vi "encodeArrayByte.vi"(8 "error in (no error)":errorcluster, 11 "Byte Array":u8[](array[numeric]) format="%.0x") -> (0 "error out":errorcluster, 3 "MessagePack":u8[](array[numeric]) format="%.0x")   [LabVIEW 2015, in "MsgPack.lvlib"]
uses:
  MsgPack.lvlib
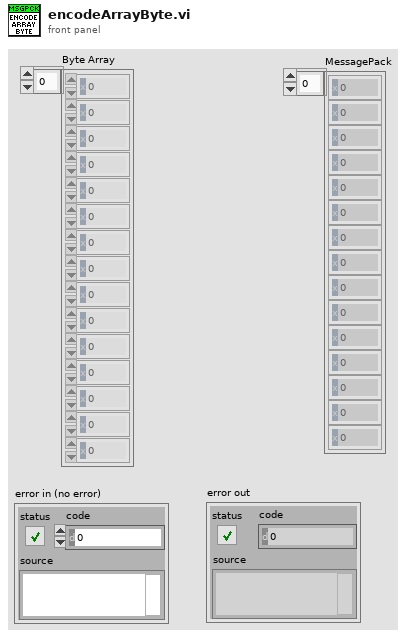
[diagram p1: front panel]
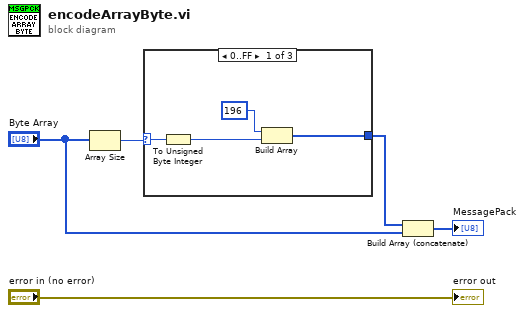
[diagram p0: block diagram]
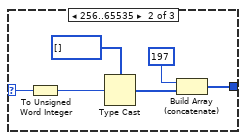
[diagram p2: hidden frame]
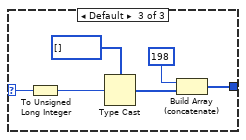
[diagram p3: hidden frame]
diagram:
  n1 = Array Size(array="Byte Array") -> (size(s)=w3:i32)
  n2 = case shown="0..FF" w3 {
    selector: w3 -> [w7 w13 w19]
    tunnel: [w8 w14 w20] -> w4
    frame 0..255 {
      n3 = To Unsigned Byte Integer(number=w7) -> (unsigned 8bit integer=w6:u8)
      n4 = Build Array(u8 196, w6) -> (w8:u8[])
    }
    frame 256..65535 {
      n5 = To Unsigned Word Integer(number=w13) -> (unsigned 16bit integer=w12:u16)
      n6 = Type Cast(type=u8[] [] ("appended array"), x=w12) -> (*(type *) &x=w10:u8[])
      n7 = Build Array (concatenate)(u8 197, w10) -> (w14:u8[])
    }
    frame Default {
      n8 = To Unsigned Long Integer(number=w19) -> (unsigned 32bit integer=w18:u32)
      n9 = Type Cast(type=u8[] [] ("appended array"), x=w18) -> (*(type *) &x=w16:u8[])
      n10 = Build Array (concatenate)(u8 198, w16) -> (w20:u8[])
    }
  }
  n11 = Build Array (concatenate)(w4, "Byte Array") -> (→"MessagePack":u8[])
  "error out" <- "error in (no error)"
